vi "Disconnect.vi"(8 "error in (no error)":errorcluster, 9 "Blocking?":bool, 10 "Timeout (5000 ms)":i32=5000, 11 "BASE.Device in":refnum<class "BASE.Device.lvclass">) -> (0 "error out":errorcluster, 3 "BASE.Device out":refnum<class "BASE.Device.lvclass">)   [LabVIEW 2019, in "BASE.Device.lvlib" / "BASE.Device.lvclass"]
uses:
  BASE.Device.lvclass
  D:/Program Files (x86)/National Instruments/LabVIEW 2019/vi.lib/ActorFramework/Actor/Actor.lvclass
  <vilib>/ActorFramework/Actor/Actor.lvclass/Actor.ctl
  <vilib>/ActorFramework/Message Enqueuer/Message Enqueuer.lvclass/Message Enqueuer.ctl
  BASE.Device Messages/Disconnect Msg/Disconnect Msg.lvclass/Disconnect Msg.ctl
  <vilib>/ActorFramework/Message Enqueuer/Init from Existing Queue.vi
  <vilib>/ActorFramework/Message Enqueuer/Enqueue.vi
  BASE.Device Messages/Disconnect Msg/Disconnect Msg.lvclass
  D:/Program Files (x86)/National Instruments/LabVIEW 2019/vi.lib/ActorFramework/Message/Message.lvclass
  <vilib>/ActorFramework/Message Priority Queue/Priority Enqueue.vi
  <vilib>/ActorFramework/Message Enqueuer/Message Enqueuer.lvclass
  <vilib>/ActorFramework/Actor/Actor.lvclass
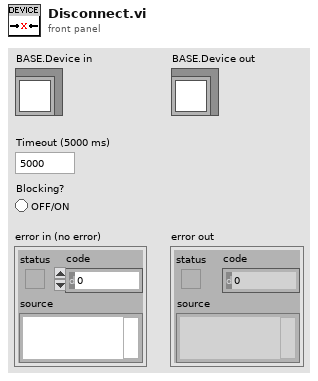
[diagram p1: front panel]
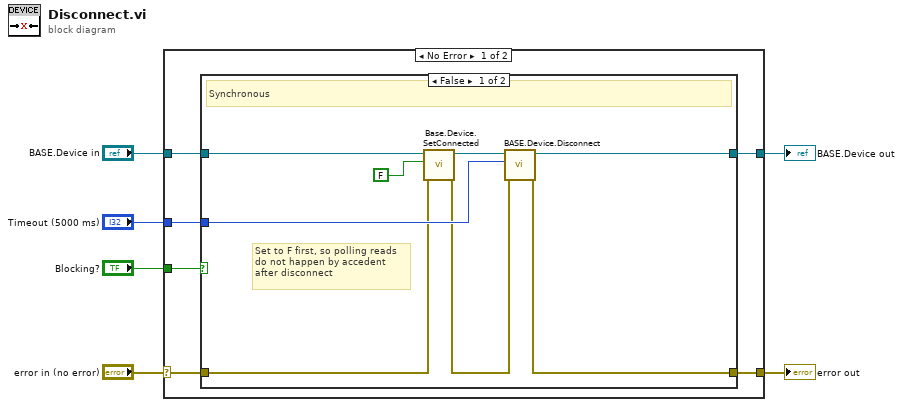
[diagram p0: block diagram]
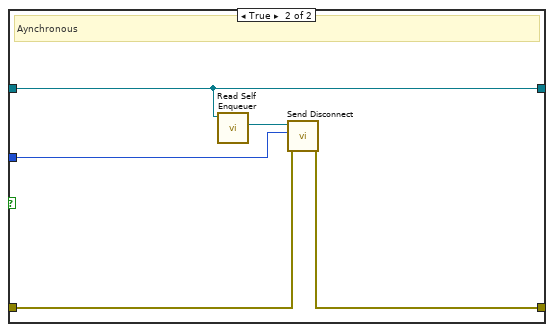
[diagram p2: hidden frame]
diagram:
  n1 = case shown="No Error" "error in (no error)" {
    selector: "error in (no error)" -> [w12 w27]
    tunnel: [w7 w27] -> w5
    tunnel: [w8 w26] -> w3
    tunnel: "BASE.Device in" -> [w9 w26]
    tunnel: "Blocking?" -> [w11 _]
    tunnel: "Timeout (5000 ms)" -> [w10 _]
    frame No Error {
      n2 = case shown="False" w11 {
        tunnel: w10 -> [w20 w23]
        tunnel: w9 -> [w17 w25]
        tunnel: [w18 w25] -> w8
        tunnel: w12 -> [w14 w22]
        tunnel: [w19 w21] -> w7
        frame False {
          # "Set to F first, so polling reads \ndo not happen by accedent \nafter disconnect"
          # "Synchronous"
          n3 = call "Base.Device.SetConnected.vi"("error in (no error)"=w14, "Connected?"=FALSE, "BASE.Device in"=w17) -> ("error out"=w13:errorcluster, "BASE.Device out"=w16:refnum<class "BASE.Device.lvclass">)  [unwired: 7 in]
          n4 = call-dynamic "BASE.Device.Disconnect.vi"("error in (no error)"=w13, "Timeout (5000 ms)"=w20, "BASE.Device in"=w16) -> ("error out"=w19:errorcluster, "BASE.Device out"=w18:refnum<class "BASE.Device.lvclass">)  [unwired: 7 in]
        }
        frame True {
          # "Aynchronous"
          n5 = call <vilib>:"Read Self Enqueuer.vi"("Actor"=w25) -> ("Self Enqueuer"=w24:refnum<class "Message Enqueuer.lvclass">)  [unwired: 10 in]
          n6 = call "Send Disconnect.vi"("error in (no error)"=w22, "Timeout (5000 ms)"=w23, "Message Enqueuer"=w24) -> ("error out"=w21:errorcluster)  [unwired: 7 in, 1 out]
        }
      }
    }
    frame Error {
    }
  }
  "error out" <- w5
  "BASE.Device out" <- w3
